vi "Test Info the Duration and Cycle Updates.vi"(8 "error in (no error)":errorcluster, 11 "Test Info in":refnum<class "Test Info.lvclass">) -> (0 "error out":errorcluster, 3 "Test Info out":refnum<class "Test Info.lvclass">)   [LabVIEW 2023, in "Data Analysis.lvlib" / "Test Info.lvlib" / "Test Info.lvclass"]
uses:
  Test Info.lvclass
  Test Info.lvclass/Test Info.ctl
  HardwareAbstractionLayer_LVOOP/Database/Database.lvclass
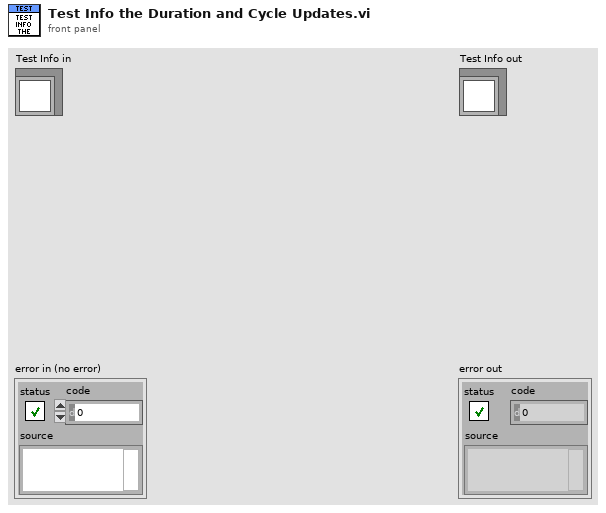
[diagram p1: front panel]
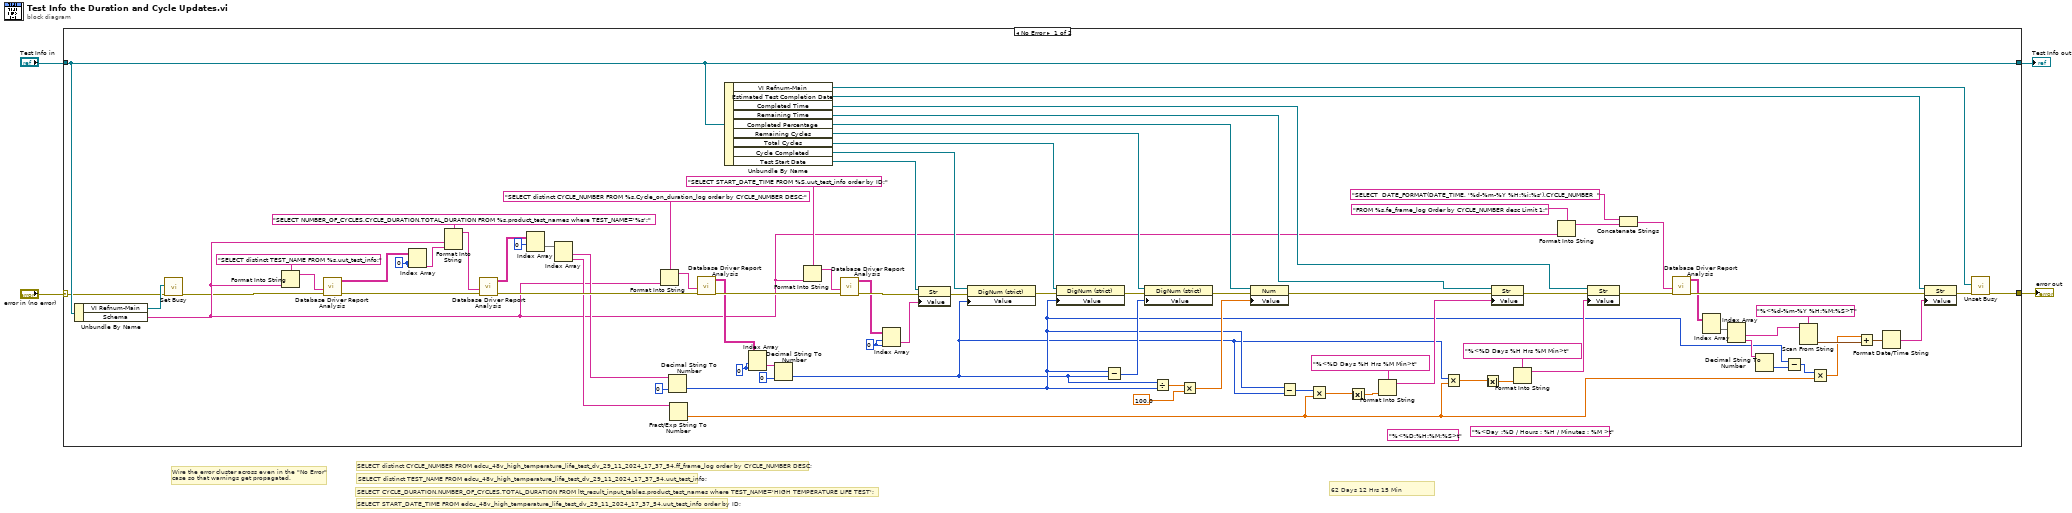
[diagram p0: block diagram]
diagram:
  # "62 Days 12 Hrs 15 Min"
  # "Wire the error cluster across even in the \"No Error\"\ncase so that warnings get propagated."
  # "SELECT START_DATE_TIME FROM edcu_48v_high_temperature_life_test_dv_29_11_2024_17_37_54.uut_test_info order by ID;"
  # "SELECT CYCLE_DURATION,NUMBER_OF_CYCLES,TOTAL_DURATION FROM ltt_result_input_tables.product_test_names where TEST_NAME='HIGH TEMPERATURE LIFE TEST';"
  # "SELECT distinct TEST_NAME FROM edcu_48v_high_temperature_life_test_dv_29_11_2024_17_37_54.uut_test_info;"
  # "SELECT distinct CYCLE_NUMBER FROM edcu_48v_high_temperature_life_test_dv_29_11_2024_17_37_54.ff_frame_log order by CYCLE_NUMBER DESC;"
  n1 = case shown="No Error" "error in (no error)" {
    selector: "error in (no error)" -> [w11 w89]
    tunnel: [w9 w89] -> w3
    tunnel: [w73 w88] -> w1
    tunnel: "Test Info in" -> [w73 w88]
    frame No Error {
      (unwired) "%<Day :%D / Hours : %H / Minutes : %M >t" ("format string")
      (unwired) "%<%D:%H:%M:%S>t" ("format string")
      w66 = 0 ("disabled index (col)")
      w69 = 0 ("disabled index (col)")
      w84 = 0 ("index (row)")
      n2 = Unbundle By Name(w73) -> ("VI Refnum-Main"=w12:refnum<vi>, "Schema"=w26:string)
      n3 = call <vilib>:"Set Busy.vi"("error in (no error)"=w11, "VI reference (current VI)"=w12) -> ("error out"=w10:errorcluster)  [unwired: 8 in, 1 out]
      n4 = Format Into String(format string="SELECT distinct TEST_NAME FROM %s.uut_test_info;", w26) -> (resulting string=w86:string)  [unwired: 2 in, 1 out]
      n5 = call "Database Driver Report Analysis.vi"("error in"=w10, "SQL query"=w86) -> ("error out"=w82:errorcluster, "data"=w85:string[][])  [unwired: 6 in, 2 out]
      n6 = Index Array(array=w85, index (row)=w84, index (col)=w84) -> (element=w33:string)
      n7 = Format Into String(format string="SELECT NUMBER_OF_CYCLES,CYCLE_DURATION,TOTAL_DURATION FROM %s.product_test_names where TEST_NAME='%s';", w26, w33) -> (resulting string=w81:string)  [unwired: 2 in, 1 out]
      n8 = call "Database Driver Report Analysis.vi"("error in"=w82, "SQL query"=w81) -> ("error out"=w79:errorcluster, "data"=w80:string[][])  [unwired: 6 in, 2 out]
      n9 = Index Array(array=w80, index (row)=0) -> (element=w60:string[])  [unwired: 1 in]
      n10 = Index Array(array=w60) -> (element #1=w59:string, element #2=w41:string)  [unwired: 2 in]
      n11 = Format Into String(format string="SELECT distinct CYCLE_NUMBER FROM %s.Cycle_on_duration_log order by CYCLE_NUMBER DESC;", w26) -> (resulting string=w77:string)  [unwired: 2 in, 1 out]
      n12 = Decimal String To Number(string=w59, default (0L)=u32 0 ("Value")) -> (number=w19:u32)  [unwired: 1 in, 1 out]
      n13 = Fract/Exp String To Number(string=w41) -> (number=w16:dbl)  [unwired: 3 in, 1 out]
      n14 = call "Database Driver Report Analysis.vi"("error in"=w79, "SQL query"=w77) -> ("error out"=w76:errorcluster, "data"=w67:string[][])  [unwired: 6 in, 2 out]
      n15 = Unbundle By Name(w73) -> ("VI Refnum-Main"=w8:refnum<vi>, "Estimated Test Completion Date"=w31:refnum<vi>, "Completed Time"=w36:refnum<vi>, "Remaining Time"=w44:refnum<vi>, "Completed Percentage"=w53:refnum<vi>, "Remaining Cycles"=w56:refnum<vi>, "Total Cycles"=w58:refnum<vi>, "Cycle Completed"=w64:refnum<vi>, "Test Start Date"=w72:refnum<vi>)
      n16 = Index Array(array=w67, index (row)=w66, index (col)=w66) -> (element=w65:string)
      n17 = Decimal String To Number(string=w65, default (0L)=u32 0 ("Value")) -> (number=w7:u32)  [unwired: 1 in, 1 out]
      n18 = Format Into String(format string="SELECT START_DATE_TIME FROM %S.uut_test_info order by ID;" ("SQL query"), w26) -> (resulting string=w74:string)  [unwired: 2 in, 1 out]
      n19 = call "Database Driver Report Analysis.vi"("error in"=w76, "SQL query"=w74) -> ("error out"=w71:errorcluster, "data"=w70:string[][])  [unwired: 6 in, 2 out]
      n20 = Index Array(array=w70, index (row)=w69, index (col)=w69) -> (element=w68:string)
      n21 = property class="Str"(reference=w72, error in=w71, "Value"=w68) -> (error out=w63:errorcluster)  [unwired: 1 out]
      n22 = property class="DigNum (strict)"(reference=w64, error in=w63, "Value"=w7) -> (error out=w57:errorcluster)  [unwired: 1 out]
      n23 = property class="DigNum (strict)"(reference=w58, error in=w57, "Value"=w19) -> (error out=w55:errorcluster)  [unwired: 1 out]
      n24 = Subtract(x=w19, y=w7) -> (x-y=w54:u32)
      n25 = property class="DigNum (strict)"(reference=w56, error in=w55, "Value"=w54) -> (error out=w52:errorcluster)  [unwired: 1 out]
      n26 = Divide(x=w7, y=w19) -> (x/y=w51:dbl)
      n27 = Multiply(x=w51, y=100.0) -> (x*y=w49:dbl)
      n28 = property class="Num"(reference=w53, error in=w52, "Value"=w49) -> (error out=w43:errorcluster)  [unwired: 1 out]
      n29 = Subtract(x=w19, y=w7) -> (x-y=w48:u32)
      n30 = Multiply(x=w48, y=w16) -> (x*y=w42:dbl)
      n31 = Absolute Value(x=w42) -> (abs(x)=w47:dbl)
      n32 = Format Into String(format string="%<%D Days %H Hrs %M Min>t", w47) -> (resulting string=w40:string)  [unwired: 2 in, 1 out]
      n33 = Multiply(x=w7, y=w16) -> (x*y=w39:dbl)
      n34 = Absolute Value(x=w39) -> (abs(x)=w37:dbl)
      n35 = property class="Str"(reference=w44, error in=w43, "Value"=w40) -> (error out=w35:errorcluster)  [unwired: 1 out]
      n36 = Format Into String(format string="%<%D Days %H Hrs %M Min>t", w37) -> (resulting string=w34:string)  [unwired: 2 in, 1 out]
      n37 = Format Into String(format string="FROM %s.fe_frame_log Order by CYCLE_NUMBER desc Limit 1;", w26) -> (resulting string=w30:string)  [unwired: 2 in, 1 out]
      n38 = property class="Str"(reference=w36, error in=w35, "Value"=w34) -> (error out=w29:errorcluster)  [unwired: 1 out]
      n39 = Concatenate Strings("SELECT  DATE_FORMAT(DATE_TIME, '%d-%m-%Y %H:%i:%s'),CYCLE_NUMBER  " ("format string"), w30) -> (w6:string)
      n40 = call "Database Driver Report Analysis.vi"("error in"=w29, "SQL query"=w6) -> ("error out"=w28:errorcluster, "data"=w25:string[][])  [unwired: 6 in, 2 out]
      n41 = Index Array(array=w25) -> (element=w24:string[])  [unwired: 2 in]
      n42 = Index Array(array=w24) -> (element #1=w22:string, element #2=w20:string)  [unwired: 2 in]
      n43 = Decimal String To Number(string=w20) -> (number=w18:i32)  [unwired: 2 in, 1 out]
      n44 = Subtract(x=w19, y=w18) -> (x-y=w17:u32)
      n45 = Scan From String(format string="%<%d-%m-%Y %H:%M:%S>T", input string=w22) -> (output 1=w21:timestamp)  [unwired: 3 in, 3 out]
      n46 = Multiply(x=w17, y=w16) -> (x*y=w15:dbl)
      n47 = Add(x=w15, y=w21) -> (x+y=w13:timestamp)
      n48 = Format Date/Time String(seconds (now)=w13) -> (date/time string=w14:string)  [unwired: 2 in]
      n49 = property class="Str"(reference=w31, error in=w28, "Value"=w14) -> (error out=w32:errorcluster)  [unwired: 1 out]
      n50 = call <vilib>:"Unset Busy.vi"("error in (no error)"=w32, "VI reference (current VI)"=w8) -> ("error out"=w9:errorcluster)  [unwired: 9 in]
    }
    frame Error {
    }
  }
  "error out" <- w3
  "Test Info out" <- w1
